vi "Get_CODE_ID.vi"(10 "PRODUCT_ID":string, 11 "CODE_MAIN":string) -> (3 "CODE_ID":string)   [LabVIEW 2020]
uses:
  Global1.vi
panel:
  out "error out":errorcluster
  in  "error in (no error)":errorcluster
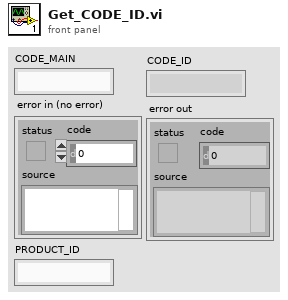
[diagram p1: front panel]
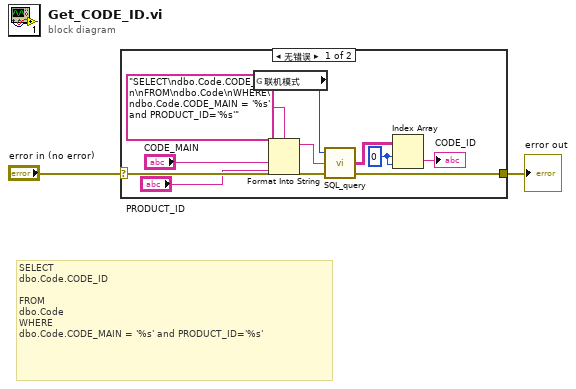
[diagram p0: block diagram]
diagram:
  # "SELECT\ndbo.Code.CODE_ID\n\nFROM\ndbo.Code\nWHERE\ndbo.Code.CODE_MAIN = '%s' and PRODUCT_ID='%s'"
  n1 = case shown="无错误" "error in (no error)" {
    selector: "error in (no error)" -> [w9 w13]
    tunnel: [w8 w13] -> w1
    frame No Error {
      w6 = 0 ("索引 (行)")
      n2 = global read "Global1.vi" "联机模式"() -> (w4:enum16{"单机", "追溯"})
      n3 = Format Into String(format string="SELECT\ndbo.Code.CODE_ID\n\nFROM\ndbo.Code\nWHERE\ndbo.Code.CODE_MAIN = '%s' and PRODUCT_ID='%s'" ("格式字符串"), "CODE_MAIN", "PRODUCT_ID") -> (resulting string=w10:string)  [unwired: 2 in, 1 out]
      n4 = call "SQL_query.vi"("error in (no error)"=w9, "SQL query"=w10, "联机模式"=w4) -> ("error out"=w8:errorcluster, "data"=w7:string[][])  [unwired: 1 out]
      n5 = Index Array(array=w7, index (row)=w6, index (col)=w6) -> (element=→"CODE_ID":string)
    }
    frame Error {
    }
  }
  "error out" <- w1
